vi "ocv.vi"(0 "IP adress":string="192.109.209.229", 1 "stop":bool, 2 "Channel":u8(ring) items=["1", "2", "3", "4", "5", "6", "7", "8", "9", "10", "11", "12", "13", "14", "15", "16"], 3 "OCV Parameters":T1={"Rest_time_T"=1.0, "Record_every_dE"=0.01, "Record_every_dT"=0.01, "E_Range"=3, "em"=1, "ce"=0, "tb"=2e-05} {"tb" min=2e-05 max=1 format="%^_3e"; "ce" items=["Standard", "CE to ground"]; "E_Range" items=["±2.5V", "±5V", "±10V", "Auto"]; "Record_every_dT" min=0 format="%.2e"; "Record_every_dE" min=0 max=100 format="%.4f"; "Rest_time_T" min=0 format="%.2f"}, 4 "Exit":bool, 5 "Start":bool, 6 "Draw":enum16{"Ewe(t)", "Ece(t)"}(ring)) -> (7 "XY Graph":cluster{"Data 100":dbl[], "Data 100":dbl[]}(graph), 8 "Number of points":i32)   [LabVIEW 2016]
doc: "The Open Circuit Voltage technique consists of a period during which no potantial or current is applied to the working electrode.\nThis VI contain others sub VIs.\nIn general,in this VI, the first thing to do is to start by establishing the connection with the instrument defined by its IP adress, then load the firmware in the channel selected, get the information on the plugged channels, load protocol on a channel, start/stop the protocol, retreive data and draw the graph."
uses:
  LLB/dll_Functions.llb/OCVParameters.ctl
panel:
  in  "Display Parameters?":bool caption="Display Parameters"
  out "DllPath":path caption="DLL Path"
  out "LibVersion":string caption="DLL Version"
  in  "Update":bool caption="Start"
  out "Exit 2":bool
  out "Data 100":dbl[][](array[numeric]) format="%.2f"
  # "Instructions:\nBefore running the VI you must type a valid IP adress that corresponds to the instrument.Then press the Run button to execute this VI.\nWhile this VI is running, choose the available channel, enter the OCV parameters or keep the default values, then press the start button to begin the experience. \nThe potential response as a function of the time (Ewe(t), Ece(t)) will be drawn."
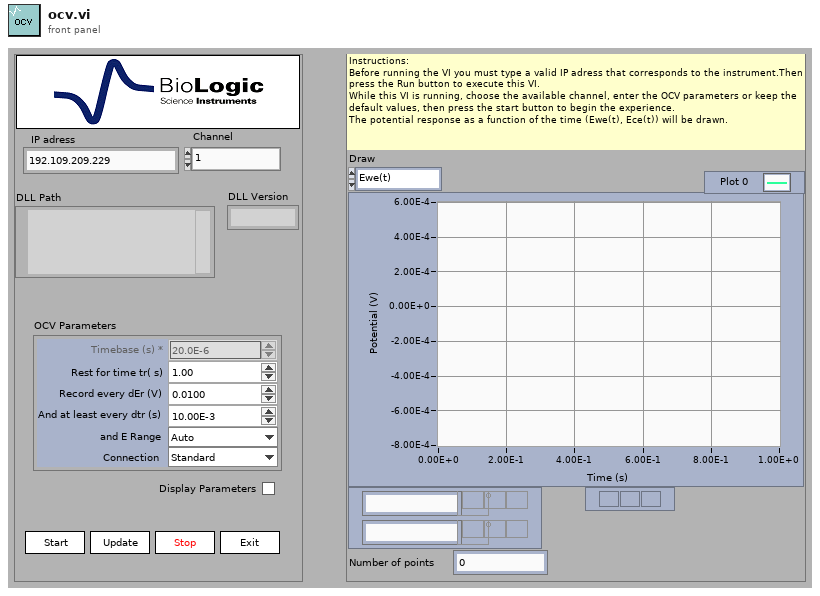
[diagram p1: front panel]
types:
  T1 = typedef "OCVParameters.ctl" = cluster{"Rest_time_T":sgl, "Record_every_dE":sgl, "Record_every_dT":sgl, "E_Range":u16, "em":u16, "ce":u16, "tb":sgl}
  T2 = cluster{"LibVersion":string, "StringLength":u32, "DllPath":path}
  T3 = typedef "TechniqueParameters.ctl" = cluster{"String Label":string, "Type":i32, "Valeur":i32, "Index":i32}
  T4 = cluster{"string before end tag":string, i32, i32, i32}[]
  T5 = cluster{"IRQskipped":i32, "NbRaws":i32, "NbCols":i32, "Technique Index":i32, "TechniqueID":i32, "PrcessIndex":i32, "loop":i32, "StartTime":dbl, "MuxPad":i32}
  T6 = cluster{"State":i32, "MemFilled":i32, "TimeBase":sgl, " Ewe":sgl, " EweRangeMin":sgl, " EweRangeMax":sgl, "Ece":sgl, "EceRangeMin":sgl, "EceRangeMax":sgl, "Eoverflow":i32, "I":sgl, "IRange":i32, "Ioverflow":i32, "ElapsedTime":sgl, "Freq":sgl, "Rcomp":sgl, "Saturation":sgl, "OptErr":i32, "OptPos":i32}
  T7 = cluster{"Rest_time_T":sgl, "Record_every_dE":sgl, "Record_every_dT":sgl, "E_Range":u16, "em":u16, "ce":u16, "tb":sgl}
  T8 = cluster{"Label":string, "type":i32, "valeur":u32, "index":i32}[]
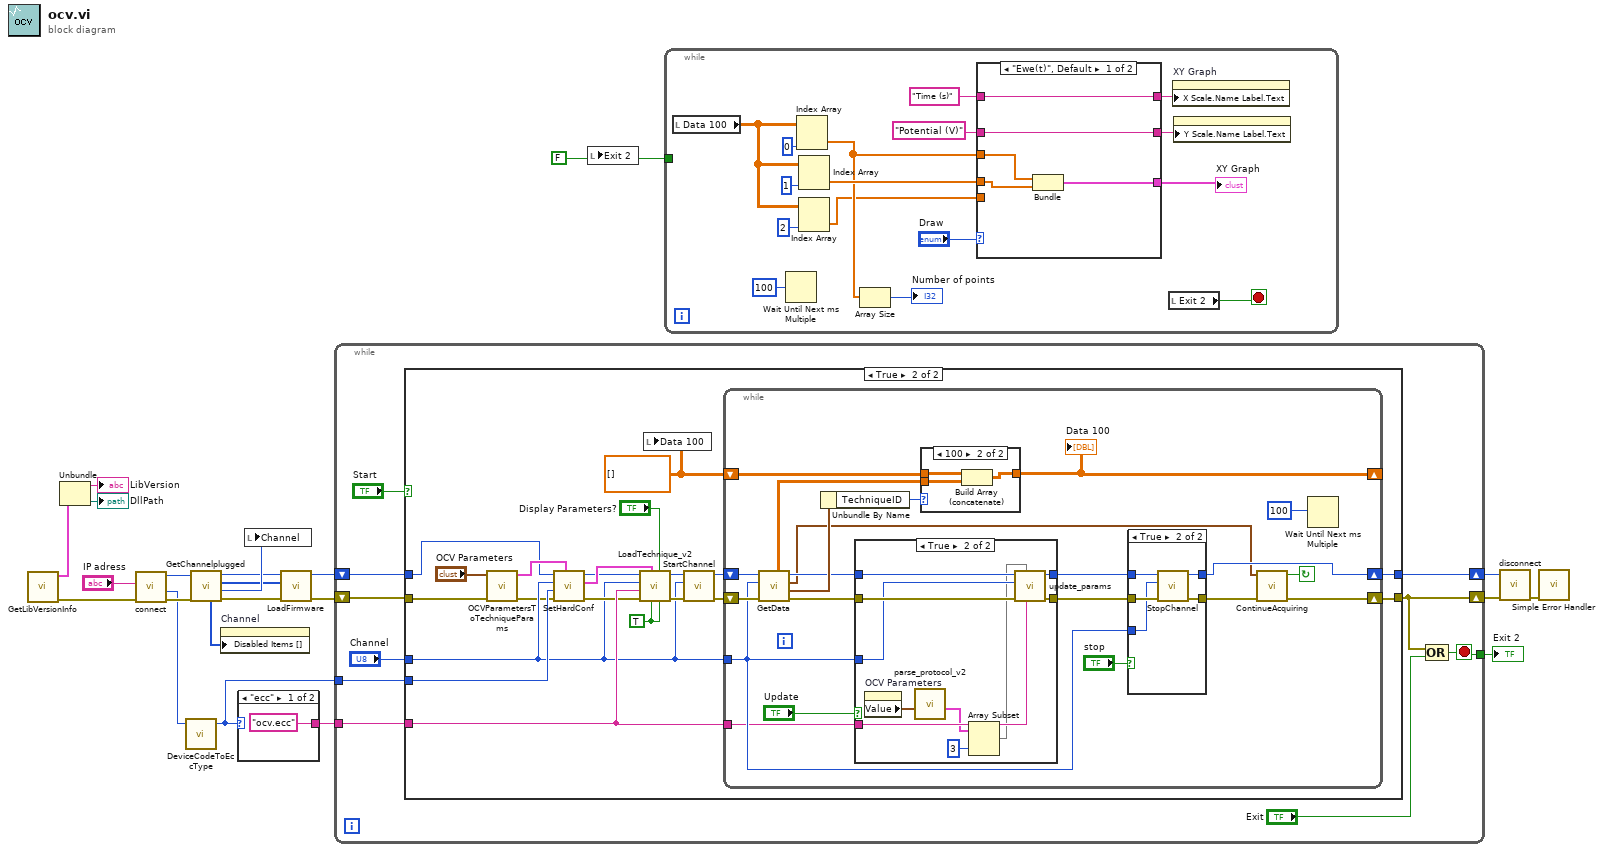
[diagram p0: block diagram]
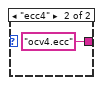
[diagram p2: hidden frame]
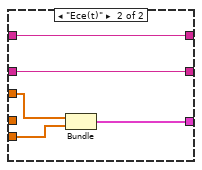
[diagram p3: hidden frame]
diagram:
  w21 = FALSE ("Exit 2")
  n1 = call "GetLibVersionInfo.vi"() -> ("error out"=w1:errorcluster, "LibInfo"=w4:T2)  [unwired: 10 in]
  n2 = Unbundle(w4) -> ("LibVersion"=→"LibVersion":string, "DllPath"=→"DllPath":path)  [unwired: 1 out]
  n3 = call "connect.vi"("error in (no error)"=w1, "IP"="IP adress") -> ("error out"=w17:errorcluster, "Device Code"=w8:i32, "ID Out"=w16:i32)  [unwired: 6 in, 1 out]
  n4 = call "DeviceCodeToEccType.vi"("Device Code"=w8) -> ("EccType"=w5:enum16{"ecc", "ecc4"})  [unwired: 4 in]
  n5 = call "GetChannelplugged.vi"("error in (no error)"=w17, "ID In"=w16) -> ("error out"=w13:errorcluster, "FirstPluggedChannel"=w19:u8, "PluggedChannels"=w12:u8[], "ID Out"=w15:i32, "DisabledChannels"=w10:i32[])  [unwired: 5 in]
  n6 = property on="Channel" class="Ring (strict)"("Disabled Items []"=w10) -> ()  [unwired: 2 in, 2 out]
  n7 = case shown="\"ecc\"" w5 {
    tunnel: ["ocv.ecc" ("FName") "ocv4.ecc" ("FName")] -> w7
    frame "ecc" {
    }
    frame "ecc4" {
    }
  }
  n8 = local write "Channel"(w19) -> ()
  n9 = call "LoadFirmware.vi"("error in (no error)"=w13, "Channels"=w12, "ID In"=w15) -> ("error out"=w11:errorcluster, "ID Out"=w14:i32)  [unwired: 6 in, 1 out]
  n10 = while {
    shift-right: [w28] -> w9
    shift-left: w11 -> [w31]
    tunnel: [w27] -> w22
    tunnel: w7 -> [w32]
    shift-right: [w34] -> w18
    shift-left: w14 -> [w30]
    tunnel: w5 -> [w26]
    stop <- w27 stop-if-true
    n11 = case shown="True" "Start" {
      tunnel: "Channel" -> [_ w41]
      tunnel: [w36 w56] -> w28
      tunnel: w31 -> [w36 w46]
      tunnel: w30 -> [w35 w39]
      tunnel: [w35 w54] -> w34
      tunnel: w32 -> [_ w52]
      tunnel: w26 -> [_ w42]
      frame False {
      }
      frame True {
        w51 = TRUE ("First Protocol")
        w55 = dbl[][] []
        n12 = call "OCVParametersToTechniqueParams.vi"("error in (no error)"=w46, "OCV Parameters"="OCV Parameters") -> ("error out"=w38:errorcluster, "TechniqueParameters"=w40:T3[])  [unwired: 8 in]
        n13 = call "SetHardConf.vi"("Params Values"=w40, "error in (no error)"=w38, "EccType"=w42, "Channel"=w41, "ID In"=w39) -> ("error out"=w43:errorcluster, "Params Values Trimed"=w45:T4, "ID Out"=w44:i32)  [unwired: 4 in]
        n14 = call "LoadTechnique_v2.vi"("Last Protocol"=w51, "Display Parameters?"="Display Parameters?", "First Protocol"=w51, "TechniqueParameters"=w45, "error in (no error)"=w43, "FName"=w52, "Selected Channel"=w41, "ID In"=w44) -> ("error out"=w47:errorcluster, "ID  Out"=w49:i32)  [unwired: 2 in]
        n15 = local write "Data 100"(w55) -> ()
        n16 = call "StartChannel.vi"("error in (no error)"=w47, "Channel"=w41, "ID In"=w49) -> ("error out"=w50:errorcluster, "ID Out"=w48:i32)  [unwired: 7 in]
        n17 = while {
          shift-right: [w60] -> w56
          shift-left: w50 -> [w77]
          shift-right: [w75] -> _
          shift-left: w55 -> [w74]
          tunnel: w41 -> [w67]
          tunnel: w52 -> [w66]
          shift-right: [w61] -> w54
          shift-left: w48 -> [w64]
          stop <- w57 continue-if-true
          n18 = call "GetData.vi"("error in (no error)"=w77, "Channel"=w67, "ID In"=w64) -> ("error out"=w69:errorcluster, "Data information"=w71:T5, "Current values"=w58:T6, "ID Out"=w62:i32, "Data"=w65:dbl[][])  [unwired: 4 in]
          n19 = Unbundle By Name(w71) -> ("TechniqueID"=w72:i32)
          n20 = case shown="True" "Update" {
            tunnel: w69 -> [w79 w89]
            tunnel: [w79 w88] -> w68
            tunnel: w62 -> [w78 w87]
            tunnel: w67 -> [_ w86]
            tunnel: w66 -> [_ w85]
            tunnel: [w78 w80] -> w63
            frame False {
            }
            frame True {
              n21 = property on="OCV Parameters" class="Clust (strict)"() -> ("Value"=w84:T7)  [unwired: 2 in, 2 out]
              n22 = call "parse_protocol_v2.vi"("Protocol Cluster"=w84) -> ("Params Values"=w83:T8)  [unwired: 10 in]
              n23 = Array Subset(array=w83, length=3) -> (w81:T8)  [unwired: 1 in]
              n24 = call "update_params.vi"("EccFileName"=w85, "Params"=w81, "error in (no error)"=w89, "Channel"=w86, "ID"=w87) -> ("error out"=w88:errorcluster, "ID Out"=w80:i32)  [unwired: 5 in]
            }
          }
          n25 = case shown="100" w72 {
            tunnel: w65 -> [_ w100]
            tunnel: [w97 w99] -> w75
            tunnel: w74 -> [w97 w98]
            frame 0, Default {
            }
            frame 100 {
              n26 = Build Array (concatenate)(w98, w100) -> (w99:dbl[][])
            }
          }
          "Data 100" <- w75
          n27 = case shown="True" "stop" {
            tunnel: [w91 w96] -> w59
            tunnel: w68 -> [w91 w95]
            tunnel: w67 -> [_ w94]
            tunnel: w63 -> [w90 w93]
            tunnel: [w90 w92] -> w61
            frame False {
            }
            frame True {
              n28 = call "StopChannel.vi"("error in (no error)"=w95, "Channel"=w94, "ID In"=w93) -> ("error out"=w96:errorcluster, "ID Out"=w92:i32)  [unwired: 7 in]
            }
          }
          n29 = call "ContinueAcquiring.vi"("error in"=w59, "Current values"=w58) -> ("error out"=w60:errorcluster, "ContinueAcquiring?"=w57:bool)  [unwired: 8 in]
          n30 = Wait Until Next ms Multiple(millisecond multiple=u32 100) -> ()  [unwired: 1 out]
        }
      }
    }
    n31 = Compound Arithmetic op=OR(w28, "Exit") -> (w27:bool)
  }
  "Exit 2" <- w22
  n32 = local write "Exit 2"(w21) -> ()
  n33 = while {
    tunnel: w21 -> [_]
    stop <- w113 stop-if-true
    n34 = local read "Data 100"() -> (w111:dbl[][])
    n35 = Wait Until Next ms Multiple(millisecond multiple=u32 100) -> ()  [unwired: 1 out]
    n36 = Index Array(array=w111, index (col)=0 ("Index")) -> (element=w104:dbl[])  [unwired: 1 in]
    n37 = Index Array(array=w111, index (col)=1 ("Index")) -> (element=w105:dbl[])  [unwired: 1 in]
    n38 = Index Array(array=w111, index (col)=2 ("indice désactivé (col)")) -> (element=w103:dbl[])  [unwired: 1 in]
    n39 = Array Size(array=w104) -> (size(s)=→"Number of points":i32)
    n40 = case shown="\"Ewe(t)\", Default" "Draw" {
      tunnel: "Time (s)" ("Y Scale.Name Label.Text") -> [w121 w126]
      tunnel: [w121 w126] -> w108
      tunnel: "Potential (V)" ("Y Scale.Name Label.Text") -> [w120 w125]
      tunnel: [w120 w125] -> w106
      tunnel: w104 -> [w119 w122]
      tunnel: w105 -> [w118 _]
      tunnel: w103 -> [_ w124]
      tunnel: [w117 w123] -> w101
      frame "Ewe(t)", Default {
        n41 = Bundle("Data 100"=w119, "Data 100"=w118) -> (w117:cluster{"Data 100":dbl[], "Data 100":dbl[]})  [unwired: 1 in]
      }
      frame "Ece(t)" {
        n42 = Bundle("Data 100"=w122, "Data 100"=w124) -> (w123:cluster{"Data 100":dbl[], "Data 100":dbl[]})  [unwired: 1 in]
      }
    }
    "XY Graph" <- w101
    n43 = local read "Exit 2"() -> (w113:bool)
    n44 = property on="XY Graph" class="XYGraph (strict)"("X Scale.Name Label.Text"=w108) -> ()  [unwired: 2 in, 2 out]
    n45 = property on="XY Graph" class="XYGraph (strict)"("Y Scale.Name Label.Text"=w106) -> ()  [unwired: 2 in, 2 out]
  }
  n46 = call "disconnect.vi"("error in (no error)"=w9, "ID In"=w18) -> ("error out"=w6:errorcluster)  [unwired: 9 in]
  n47 = call <vilib>:"Simple Error Handler.vi"("error in (no error)"=w6) -> ()  [unwired: 4 in, 5 out]
